vi "Configure Correction.vi"(7 "Enable Correction (T: Enable)":bool=TRUE, 8 "error in (no error)":errorcluster, 9 "Cal Type (\"Full 2 Port with power(1,2)\")":string="Full 2 Port with power(1,2)", 10 "Channel (1)":i32=1, 11 "VISA resource name":refnum<visa-resource-name>) -> (0 "error out":errorcluster, 3 "VISA resource name out":refnum<visa-resource-name>)   [LabVIEW 2018, in "Keysight PNA Series.lvlib"]
doc: "Configures error correction for the selected measurement on the specified channel."
uses:
  Keysight PNA Series.lvlib
panel:
  # "TODO:\nThis VI still has problem."
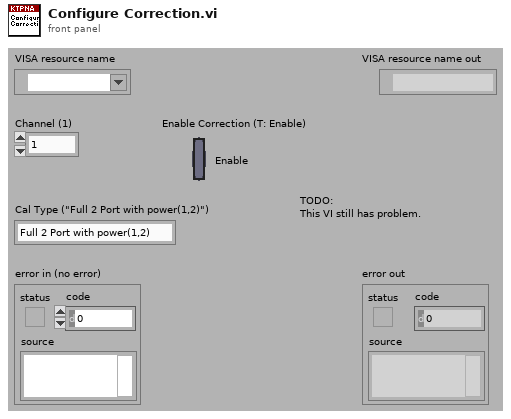
[diagram p1: front panel]
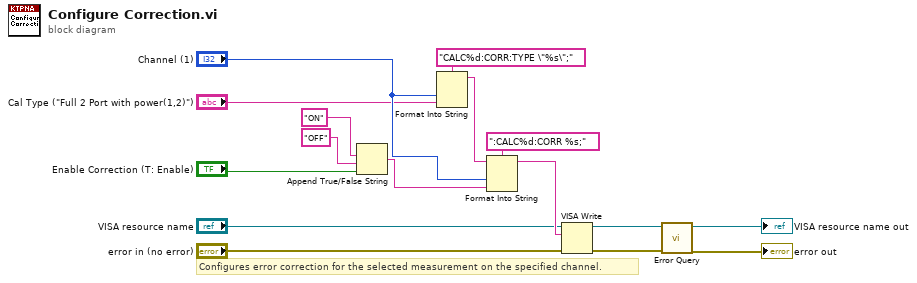
[diagram p0: block diagram]
diagram:
  # "Configures error correction for the selected measurement on the specified channel."
  n1 = Append True/False String(1:"Enable Correction (T: Enable)", 2:"OFF", 3:"ON") -> (0:w8:string)  [unwired: 1 in]
  n2 = Format Into String(format string="CALC%d:CORR:TYPE \"%s\";", "Channel (1)", "Cal Type (\"Full 2 Port with power(1,2)\")") -> (resulting string=w10:string)  [unwired: 2 in, 1 out]
  n3 = Format Into String(format string=":CALC%d:CORR %s;", initial string=w10, "Channel (1)", w8) -> (resulting string=w7:string)  [unwired: 1 in, 1 out]
  n4 = VISA Write(VISA resource name="VISA resource name", write buffer=w7, error in (no error)="error in (no error)") -> (VISA resource name out=w1:refnum<visa-resource-name>, error out=w4:errorcluster)  [unwired: 1 out]
  n5 = call "Error Query.vi"("error in (no error)"=w4, "VISA resource name"=w1) -> ("error out"=→"error out":errorcluster, "VISA resource name out"=→"VISA resource name out":refnum<visa-resource-name>)  [unwired: 6 in, 2 out]
